vi "RT Main.vi"() -> ()   [LabVIEW 2017]
uses:
  <vilib>/NI/Module Execution Interface/Engine Runtime/Execution States.ctl
  <vilib>/NI/Module Execution Interface/Engine Runtime/Fault.ctl
  <vilib>/NI/Tag Bus Module Framework/runtime/error classification.ctl
  <vilib>/NI/Module Execution Interface/Engine Runtime/Engine Runtime Interface.lvclass
  <vilib>/NI/Tag Bus Module Framework/runtime/TBM module execution interface.lvclass
  <vilib>/NI/DCAF/Tag Editor Core/Framework Configuration Classes/target runtime/PL_Target Runtime.lvclass
  <vilib>/NI/Tag Bus Module Framework/FPGA manager/methods.ctl
  <vilib>/NI/Tag Bus Module Framework/FPGA manager/FPGA manager.lvlib
panel:
  out "error out":errorcluster
  in  "configuration file path":path=path "/home/lvuser/ExecTemplate.pcfg"
  in  "target alias":string="IC"
  in  "Engine_Stop":bool
  out "engine status":T4(array[cluster])
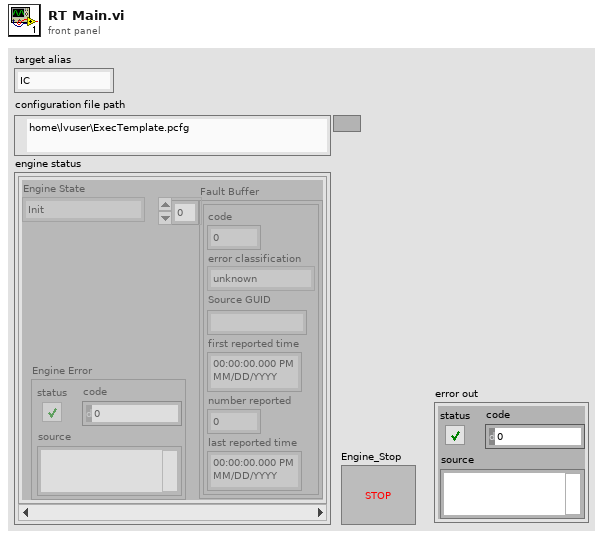
[diagram p1: front panel]
types:
  T1 = typedef "Engine Runtime Interface.lvclass/Execution States.ctl" = enum16{"Init", "Pre-Operational", "Safe-Operational", "Operational", "Stopped"}
  T2 = typedef "Engine Runtime Interface.lvclass/Fault.ctl" = cluster{"code":i32, "error classification":T3, "Source GUID":string, "first reported time":timestamp, "number reported":u32, "last reported time":timestamp}
  T3 = typedef "TBM module execution interface.lvclass/error classification.ctl" = enum16{"unknown", "none", "trivial", "recoverable", "critical"}
  T4 = cluster{"Engine State":T1, "Fault Buffer":T2[], "Engine Error":errorcluster}[]
  T5 = cluster{"Engine State":T1, "Fault Buffer":T2[], "Engine Error":errorcluster}
  T6 = typedef "FPGA manager.lvlib/methods.ctl" = enum16{"initialize bitfile", "cache bitfile", "locate bitfile", "close bitfile", "clear manager"}
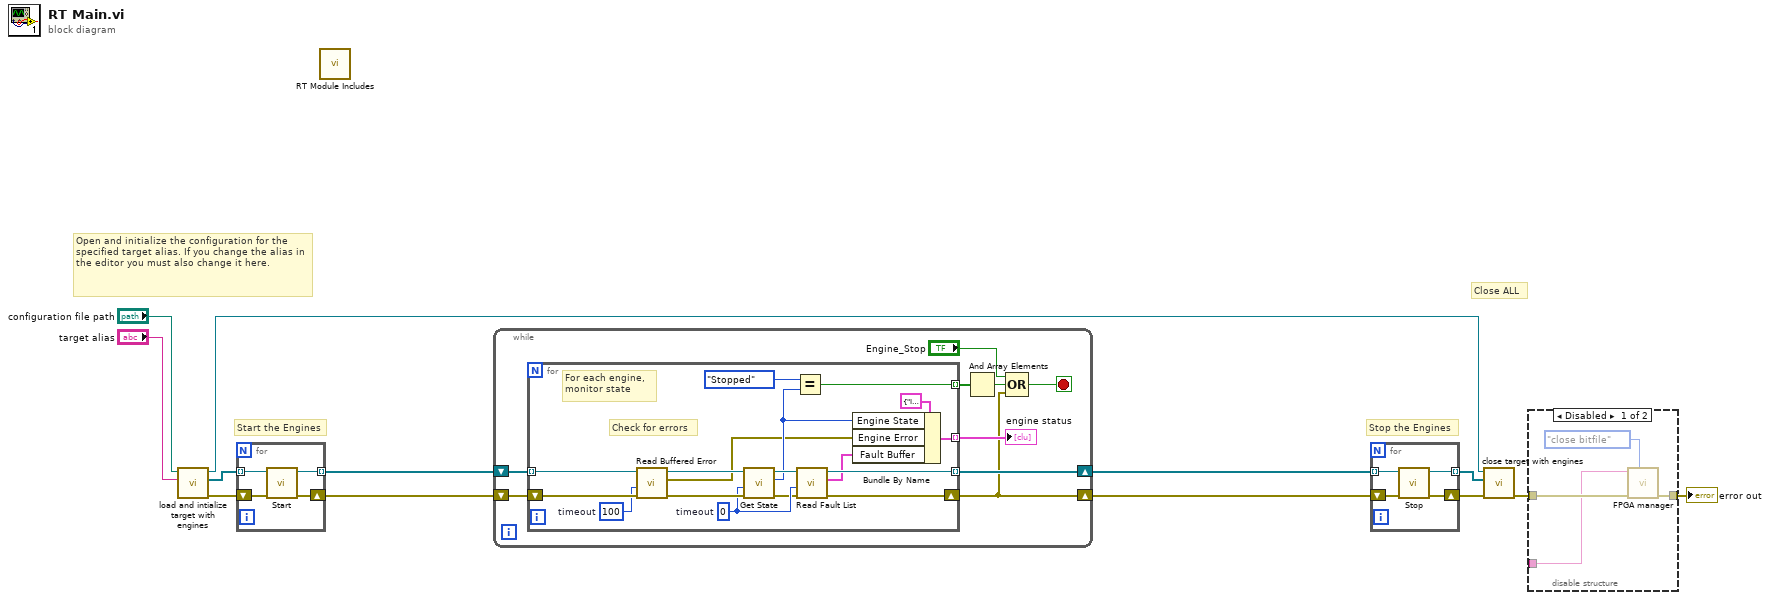
[diagram p0: block diagram]
diagram:
  # "Start the Engines"
  # "Open and initialize the configuration for the specified target alias. If you change the alias in the editor you must also change it here."
  # "Close ALL"
  # "Stop the Engines"
  n1 = call <vilib>:"load and intialize target with engines.vi"("target alias"="target alias", "file path"="configuration file path") -> ("error out"=w10:errorcluster, "engine runtime interfaces"=w9:refnum<class "Engine Runtime Interface.lvclass">[], "target runtime"=w6:refnum<class "PL_Target Runtime.lvclass">)  [unwired: 7 in]
  n2 = for {
    tunnel: [w17] -> w13 mode=indexing
    tunnel: w9 -> [w14] mode=indexing
    shift-right: [w16] -> w2
    shift-left: w10 -> [w15]
    n3 = call-dynamic "Start.vi"("error in"=w15, "Engine Runtime Interface in"=w14) -> ("error out"=w16:errorcluster, "Engine Runtime Interface out"=w17:refnum<class "Engine Runtime Interface.lvclass">)  [unwired: 8 in]
  }
  n4 = call "RT Module Includes.vi"() -> ()  [unwired: 12 in]
  n5 = while {
    shift-right: [w24] -> w12
    shift-left: w13 -> [w26]
    shift-right: [w18] -> w11
    shift-left: w2 -> [w25]
    stop <- w22 stop-if-true
    n6 = for {
      tunnel: w26 -> [w43] mode=indexing
      tunnel: [w35] -> w24 mode=indexing
      tunnel: [w38] -> w20 mode=indexing
      shift-right: [w34] -> w18
      shift-left: w25 -> [w42]
      tunnel: [w30] -> w21 mode=indexing
      w33 = 0  # timeout
      w37 = 100  # timeout
      # "For each engine, \nmonitor state"
      # "Check for errors"
      n7 = call-dynamic "Read Buffered Error.vi"("error in"=w42, "timeout in ms (0)"=w37, "Engine Runtime Interface in"=w43) -> ("error out"=w40:errorcluster, "Engine Error"=w28:errorcluster, "Engine Runtime Interface out"=w41:refnum<class "Engine Runtime Interface.lvclass">)  [unwired: 6 in]
      n8 = call-dynamic "Get State.vi"("error in"=w40, "timeout (-1)"=w33, "Engine Runtime Interface in"=w41) -> ("error out"=w27:errorcluster, "Engine State"=w32:T1, "Engine Runtime Interface out"=w36:refnum<class "Engine Runtime Interface.lvclass">)  [unwired: 6 in]
      n9 = Equal?(x=Execution_States."Stopped" ("Engine State"), y=w32) -> (x = y?=w38:bool)
      n10 = call-dynamic "Read Fault List.vi"("error in"=w27, "timeout (-1)"=w33, "Engine Runtime Interface in"=w36) -> ("error out"=w34:errorcluster, "faults"=w31:T2[], "Engine Runtime Interface out"=w35:refnum<class "Engine Runtime Interface.lvclass">)  [unwired: 6 in]
      n11 = Bundle By Name(cluster=T5 {"Engine State"=enum."Init", "Fault Buffer"=[], "Engine Error"={"status"=FALSE, "code"=0, "source"=""}}, "Engine State"=w32, "Engine Error"=w28, "Fault Buffer"=w31) -> (w30:T5)
    }
    "engine status" <- w21
    n12 = And Array Elements(Boolean array=w20) -> (logical AND=w19:bool)
    n13 = Compound Arithmetic op=OR("Engine_Stop", w19, w18) -> (w22:bool)
  }
  n14 = for {
    tunnel: w12 -> [w47] mode=indexing
    shift-right: [w44] -> w5
    shift-left: w11 -> [w46]
    tunnel: [w45] -> w7 mode=indexing
    n15 = call-dynamic "Stop.vi"("error in"=w46, "Engine Runtime Interface in"=w47) -> ("error out"=w44:errorcluster, "Engine Runtime Interface out"=w45:refnum<class "Engine Runtime Interface.lvclass">)  [unwired: 8 in]
  }
  n16 = call <vilib>:"close target with engines.vi"("error in"=w5, "Engine Runtime Interfaces"=w7, "Target Runtime"=w6) -> ("error out"=w3:errorcluster)  [unwired: 8 in]
  n17 = disable-structure shown="Disabled" {
    disable-tunnel: [w50 w52] -> w1
    disable-tunnel: w3 -> [w51 w52]
    disable-tunnel: _ -> [w48 _]
    frame Disabled {
      n18 = call <vilib>:"FPGA manager.vi"("action"=methods."close bitfile", "error in"=w51, "RIO resource"=w48) -> ("error out"=w50:errorcluster)  [unwired: 6 in, 2 out]
    }
    frame Enabled {
    }
  }
  "error out" <- w1
